vi "LV SciSDK RATEMETER.vi"(8 "error in (no error)":errorcluster, 9 "Ratemeter Handle In":T2) -> (0 "error out":errorcluster, 1 "Ratemeter Handle Out":T2, 2 "buffer out":T1)   [LabVIEW 2021]
uses:
  SciSDK_Labview.lvlib
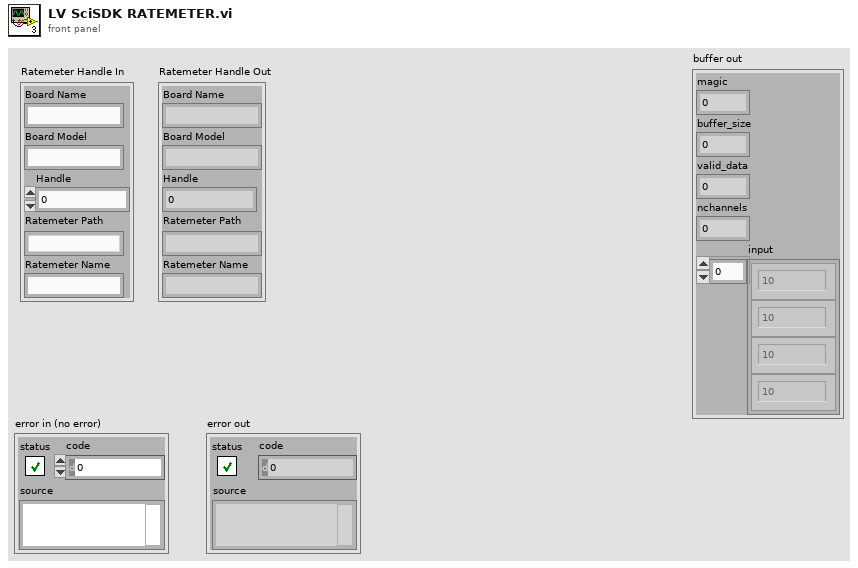
[diagram p1: front panel]
types:
  T1 = cluster{"magic":u32, "buffer_size":u32, "valid_data":u32, "nchannels":u32, "input":u32[]}
  T2 = cluster{"Board Name":string, "Board Model":string, "Handle":u64, "Ratemeter Path":string, "Ratemeter Name":string}
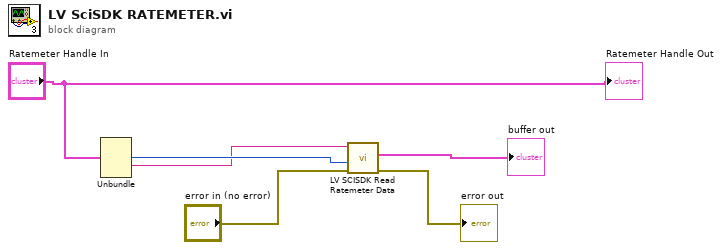
[diagram p0: block diagram]
diagram:
  n1 = Unbundle("Ratemeter Handle In") -> ("Handle"=w5:u64, "Ratemeter Path"=w4:string)  [unwired: 3 out]
  n2 = call "LV SCISDK Read Ratemeter Data.vi"("Path"=w4, "handle"=w5, "error in (no error)"="error in (no error)") -> ("buffer out"=→"buffer out":T1, "error out"=→"error out":errorcluster)  [unwired: 4 in, 2 out]
  "Ratemeter Handle Out" <- "Ratemeter Handle In"
